vi "Read Light Select.vi"(8 "error in (no error)":errorcluster, 11 "Light Stack in":refnum<class "Light Stack.lvclass">) -> (0 "error out":errorcluster, 2 "Light Select":T1, 3 "Light Stack out":refnum<class "Light Stack.lvclass">)   [LabVIEW 2018, in "Light Stack.lvlib" / "Light Stack.lvclass"]
uses:
  Light Stack.lvclass
  Custom Controls/Light Select.ctl
  Light Stack.lvclass/Light Stack.ctl
  Light Stack.lvlib
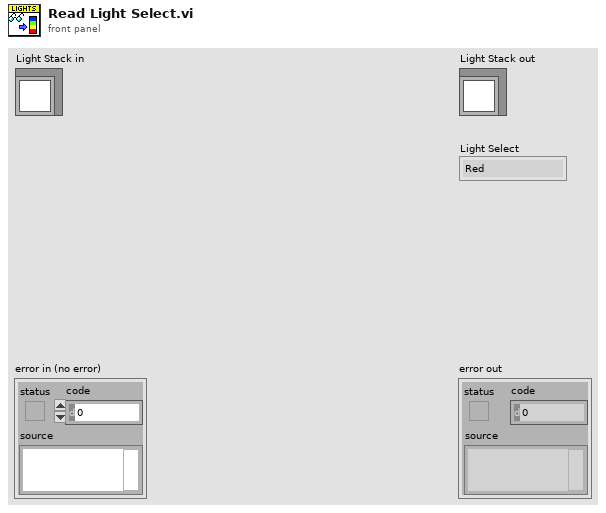
[diagram p1: front panel]
types:
  T1 = typedef "Light Stack.lvlib/Light Select.ctl" = enum16{"Red", "Amber", "Green", "Blue"}
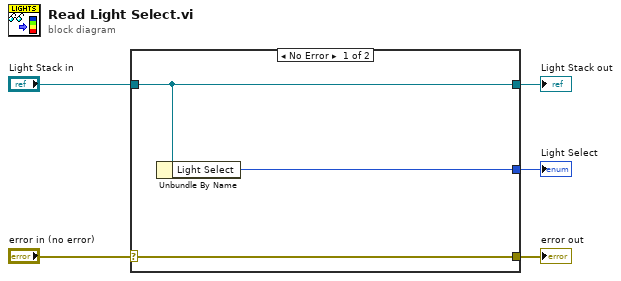
[diagram p0: block diagram]
diagram:
  n1 = case shown="No Error" "error in (no error)" {
    selector: "error in (no error)" -> [w8 w9]
    tunnel: [w8 w9] -> w4
    tunnel: [w7 w10] -> w2
    tunnel: "Light Stack in" -> [w7 w10]
    tunnel: [w6 _] -> w1
    frame No Error {
      n2 = Unbundle By Name(w7) -> ("Light Select"=w6:T1)
    }
    frame Error {
    }
  }
  "error out" <- w4
  "Light Stack out" <- w2
  "Light Select" <- w1
